vi "Pulse Attribute, Get Input Parms.vi"(5 "labels":string[](array[string])=["Number of Samples", "Sample Frequency (MHz)", "dt (us)", "Resistance (ohms)", "Average Size"], 6 "error in":errorcluster, 9 "waveform":waveform(dbl)={"t0"=timestamp(3473168073.631 s since 1904-01-01), "dt"=1e-08, "Y"=[], "attributes"=variant("Average Size"=variant(dbl 15.0), "Frequency (Hz)"=variant(dbl 1998.0127546741205), "MD5[0]"=variant(dbl 3432209604.0), "MD5[1]"=variant(dbl 1216260660.0), "MD5[2]"=variant(dbl 1007192998.0), "MD5[3]"=variant(dbl 1264973305.0), "NSamp"=variant(dbl 400000.0), "Number of Samples"=variant(dbl 400000.0), "Process Timestamp"=variant(timestamp timestamp(3474391892.1875 s since 1904-01-01)), "Recvy Amp (V)"=variant(dbl 2.6382379145344714), "Recvy Amp (mA)"=variant(dbl 5.276475829068943), "Recvy Frequency (Hz)"=variant(dbl 1998.1571037522094), "Recvy Pulse Width (us)"=variant(dbl 12.432430276870729), "Recvy Trigger (s)"=variant(dbl 0.00044008000000000003), "Resistance (ohms)"=variant(dbl 500.0), "Samp Freq (MHz)"=variant(dbl 100.0), "Sample Freq (MHz)"=variant(dbl 100.0), "Stim Amp (V)"=variant(dbl -2.3035646134631413), "Stim Amp (mA)"=variant(dbl -4.607129226926283), "Stim Frequency (Hz)"=variant(dbl 1997.8684055960314), "Stim Pulse Width (us)"=variant(dbl 12.07493911743164), "Stim Trigger (s)"=variant(dbl 0.00041221), "dt (us)"=variant(dbl 0.01))}) -> (0 "error out":errorcluster, 3 "waveform dup":waveform(dbl)={"t0"=timestamp(-9593225999.369 s since 1904-01-01), "dt"=nan, "Y"=[], "attributes"=variant("Average Size"=variant(dbl 15.0), "Frequency (Hz)"=variant(dbl 1997.9906429610444), "NSamp"=variant(dbl 400000.0), "Recvy Amp (mA)"=variant(dbl 5.267865023873527), "Recvy Amp (mV)"=variant(dbl 2633.932511936763), "Recvy Frequency (Hz)"=variant(dbl 1998.1395072914302), "Recvy Pulse Width (us)"=variant(dbl 12.427603778839112), "Recvy Trigger (s)"=variant(dbl 0.00043972), "Resistance (ohms)"=variant(dbl 500.0), "Samp Freq (MHz)"=variant(dbl 100.0), "Stim Amp (mA)"=variant(dbl -4.607747165232184), "Stim Amp (mV)"=variant(dbl -2303.873582616092), "Stim Frequency (Hz)"=variant(dbl 1997.8417786306586), "Stim Pulse Width (us)"=variant(dbl 12.076313257217407), "Stim Trigger (s)"=variant(dbl 0.00041185), "dt (us)"=variant(dbl 0.01))}, 4 "input parameters":T1[](array[typedef]) {"Value" format="%#.3f"})   [LabVIEW 2010]
doc: "This function extracts Input Parameters from the waveform attributes."
uses:
  Generic/Waveform Attribute/Waveform Attribute Cluster.ctl
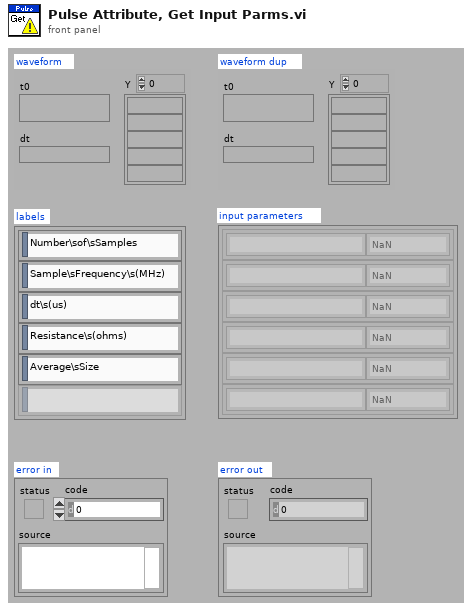
[diagram p1: front panel]
types:
  T1 = typedef "Waveform Attribute Cluster.ctl" = cluster{"Label":string, "Value":dbl}
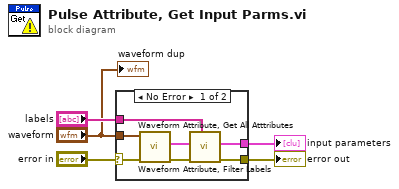
[diagram p0: block diagram]
diagram:
  n1 = case shown="No Error" "error in" {
    selector: "error in" -> [w10 w13]
    tunnel: "labels" -> [w7 _]
    tunnel: [w9 w13] -> w3
    tunnel: [w8 _] -> w2
    tunnel: "waveform" -> [w6 _]
    frame No Error {
      n2 = call "Waveform Attribute, Get All Atttributes.vi"("error in"=w10, "waveform"=w6) -> ("error out"=w12:errorcluster, "all attributes"=w11:T1[])  [unwired: 5 in, 1 out]
      n3 = call "Waveform Attribute, Filter Labels.vi"("labels"=w7, "error in"=w12, "attributes"=w11) -> ("error out"=w9:errorcluster, "filtered results"=w8:T1[])  [unwired: 5 in]
    }
    frame Error {
    }
  }
  "input parameters" <- w2
  "error out" <- w3
  "waveform dup" <- "waveform"
